vi "ServerReflection ServerReflectionInfo Read.vi"(8 "error in":errorcluster, 11 "Call ID in":T3) -> (0 "error out":errorcluster, 1 "Success":bool, 2 "Response Data":T1, 3 "Call ID":T3)   [LabVIEW 2025, in "reflection_client.lvlib"]
uses:
  reflection_client.lvlib
  <vilib>/gRPC/LabVIEW gRPC Library/Shared/grpcId.ctl
  RPC Messages/grpc_reflection_v1alpha_ServerReflectionResponse.ctl
  RPC Messages/grpc_reflection_v1alpha_ServerReflectionRequest_message_request/grpc_reflection_v1alpha_ServerReflectionRequest_message_request.lvclass
  RPC Messages/grpc_reflection_v1alpha_ServerReflectionResponse_message_response/grpc_reflection_v1alpha_ServerReflectionResponse_message_response.lvclass
  RPC Messages/grpc_reflection_v1alpha_ServerReflectionRequest.ctl
  RPC Messages/grpc_reflection_v1alpha_ServerReflectionResponse_Flat.ctl
  RPC Messages/grpc_reflection_v1alpha_ServerReflectionRequest_Flat.ctl
  RPC Messages/grpc_reflection_v1alpha_ExtensionRequest_Flat.ctl
  RPC Messages/grpc_reflection_v1alpha_FileDescriptorResponse_Flat.ctl
  RPC Messages/grpc_reflection_v1alpha_ExtensionNumberResponse_Flat.ctl
  RPC Messages/grpc_reflection_v1alpha_ListServiceResponse_Flat.ctl
  RPC Messages/grpc_reflection_v1alpha_ServiceResponse_Flat.ctl
  RPC Messages/grpc_reflection_v1alpha_ErrorResponse_Flat.ctl
  RPC Messages/grpc_reflection_v1alpha_ServerReflectionRequest_message_request/grpc_reflection_v1alpha_ServerReflectionRequest_message_request.lvclass/grpc_reflection_v1alpha_ServerReflectionRequest_message_request.ctl
  RPC Messages/grpc_reflection_v1alpha_ServerReflectionResponse_message_response/grpc_reflection_v1alpha_ServerReflectionResponse_message_response.lvclass/grpc_reflection_v1alpha_ServerReflectionResponse_message_response.ctl
  aea5dbbb-03a2-479b-ad95-94da4ee1cea9.vi
  <vilib>/gRPC/LabVIEW gRPC Library/Shared/TranslateGrpcError.vi
  <vilib>/gRPC/LabVIEW gRPC Library/Shared/Wait On Occurrence.vi
  RPC Messages/FlatToRichgrpc_reflection_v1alpha_ServerReflectionRequest.vi
  RPC Messages/grpc_reflection_v1alpha_ServerReflectionResponse_message_response/Setfile_descriptor_response.vi
  RPC Messages/FlatToRichgrpc_reflection_v1alpha_FileDescriptorResponse.vi
  RPC Messages/grpc_reflection_v1alpha_ServerReflectionResponse_message_response/Setall_extension_numbers_response.vi
  RPC Messages/FlatToRichgrpc_reflection_v1alpha_ExtensionNumberResponse.vi
  RPC Messages/grpc_reflection_v1alpha_ServerReflectionResponse_message_response/Setlist_services_response.vi
  RPC Messages/FlatToRichgrpc_reflection_v1alpha_ListServiceResponse.vi
  RPC Messages/grpc_reflection_v1alpha_ServerReflectionResponse_message_response/Seterror_response.vi
  RPC Messages/FlatToRichgrpc_reflection_v1alpha_ErrorResponse.vi
  <vilib>/gRPC/LabVIEW gRPC Library/Shared/Is Feature Enabled.vi
  RPC Messages/grpc_reflection_v1alpha_ServerReflectionRequest_message_request/Setfile_by_filename.vi
  RPC Messages/grpc_reflection_v1alpha_ServerReflectionRequest_message_request/Setfile_containing_symbol.vi
  RPC Messages/grpc_reflection_v1alpha_ServerReflectionRequest_message_request/Setfile_containing_extension.vi
  RPC Messages/FlatToRichgrpc_reflection_v1alpha_ExtensionRequest.vi
  RPC Messages/grpc_reflection_v1alpha_ServerReflectionRequest_message_request/Setall_extension_numbers_of_type.vi
  RPC Messages/grpc_reflection_v1alpha_ServerReflectionRequest_message_request/Setlist_services.vi
  RPC Messages/FlatToRichgrpc_reflection_v1alpha_ServiceResponse.vi
  <vilib>/gRPC/LabVIEW gRPC Library/Server API/Server/Get Server DLL Path.vi
  <vilib>/Utility/error.llb/Error Cluster From Error Code.vi
  RPC Messages/grpc_reflection_v1alpha_ServerReflectionResponse_message_response/GetActiveFieldName.vi
  RPC Messages/grpc_reflection_v1alpha_ServerReflectionRequest_message_request/GetActiveFieldName.vi
  <vilib>/gRPC/LabVIEW gRPC Library/grpc-lvsupport-release.lvlib
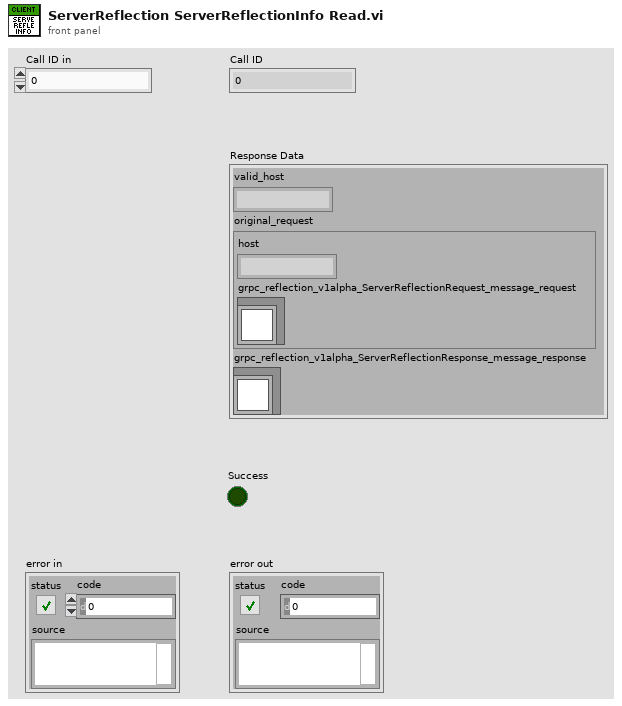
[diagram p1: front panel]
types:
  T1 = typedef "reflection_client.lvlib/grpc_reflection_v1alpha_ServerReflectionResponse.ctl" = cluster{"valid_host":string, "original_request":T2, "grpc_reflection_v1alpha_ServerReflectionResponse_message_response":refnum<class "grpc_reflection_v1alpha_ServerReflectionResponse_message_response.lvclass">}
  T2 = typedef "reflection_client.lvlib/grpc_reflection_v1alpha_ServerReflectionRequest.ctl" = cluster{"host":string, "grpc_reflection_v1alpha_ServerReflectionRequest_message_request":refnum<class "grpc_reflection_v1alpha_ServerReflectionRequest_message_request.lvclass">}
  T3 = typedef "grpc-lvsupport-release.lvlib/grpcId.ctl" = u64
  T4 = typedef "reflection_client.lvlib/grpc_reflection_v1alpha_ServerReflectionResponse_Flat.ctl" = cluster{"valid_host":string, "original_request":T5, "grpc_reflection_v1alpha_ServerReflectionResponse_message_response_selected_index":i32, "file_descriptor_response":T7, "all_extension_numbers_response":T8, "list_services_response":T9, "error_response":T11}
  T5 = typedef "reflection_client.lvlib/grpc_reflection_v1alpha_ServerReflectionRequest_Flat.ctl" = cluster{"host":string, "grpc_reflection_v1alpha_ServerReflectionRequest_message_request_selected_index":i32, "file_by_filename":string, "file_containing_symbol":string, "file_containing_extension":T6, "all_extension_numbers_of_type":string, "list_services":string}
  T6 = typedef "reflection_client.lvlib/grpc_reflection_v1alpha_ExtensionRequest_Flat.ctl" = cluster{"containing_type":string, "extension_number":i32}
  T7 = typedef "reflection_client.lvlib/grpc_reflection_v1alpha_FileDescriptorResponse_Flat.ctl" = cluster{"file_descriptor_proto":cluster{"Array":u8[]}[]}
  T8 = typedef "reflection_client.lvlib/grpc_reflection_v1alpha_ExtensionNumberResponse_Flat.ctl" = cluster{"base_type_name":string, "extension_number":i32[]}
  T9 = typedef "reflection_client.lvlib/grpc_reflection_v1alpha_ListServiceResponse_Flat.ctl" = cluster{"service":T10[]}
  T10 = typedef "reflection_client.lvlib/grpc_reflection_v1alpha_ServiceResponse_Flat.ctl" = cluster{"name":string}
  T11 = typedef "reflection_client.lvlib/grpc_reflection_v1alpha_ErrorResponse_Flat.ctl" = cluster{"error_code":i32, "error_message":string}
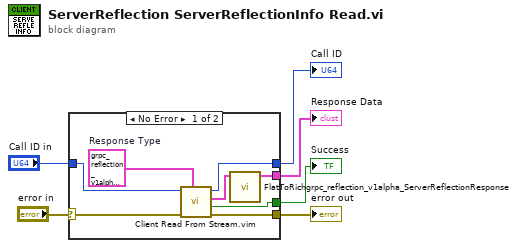
[diagram p0: block diagram]
diagram:
  n1 = case shown="No Error" "error in" {
    selector: "error in" -> [w14 w15]
    tunnel: [w13 w15] -> w5
    tunnel: "Call ID in" -> [w12 w16]
    tunnel: [w10 w16] -> w3
    tunnel: [w7 _] -> w2
    tunnel: [w11 _] -> w1
    frame No Error {
      w9 = T4 {"valid_host"="", "original_request"={"host"="", "grpc_reflection_v1alpha_ServerReflectionRequest_message_request_selected_index"=0, "file_by_filename"="", "file_containing_symbol"="", "file_containing_extension"={"containing_type"="", "extension_number"=0}, "all_extension_numbers_of_type"="", "list_services"=""}, "grpc_reflection_v1alpha_ServerReflectionResponse_message_response_selected_index"=0, "file_descriptor_response"={"file_descriptor_proto"=[]}, "all_extension_numbers_response"={"base_type_name"="", "extension_number"=[]}, "list_services_response"={"service"=[]}, "error_response"={"error_code"=0, "error_message"=""}}  # Response Type
      n2 = call "Client Read From Stream.vim"("Response Type"=w9, "error in"=w14, "Call ID in"=w12) -> ("error out"=w13:errorcluster, "Success"=w11:bool, "Response Data"=w8:T4, "Call ID out"=w10:u64)  [unwired: 5 in]
      n3 = call "FlatToRichgrpc_reflection_v1alpha_ServerReflectionResponse.vi"("InputCluster"=w8) -> ("OutputCluster"=w7:T1)  [unwired: 10 in]
    }
    frame Error {
    }
  }
  "error out" <- w5
  "Call ID" <- w3
  "Response Data" <- w2
  "Success" <- w1
